vi "MOKO Graph.vi"() -> ()   [LabVIEW 2018]
uses:
  Lib/STM/Graph/MOKO_Graph_main_STM.ctl
  Lib/STM/Graph/MOKO_Graph_main_ITEM.ctl
  Lib/STM/Grafic/MOKO_Grafic_ITEM.ctl
  Lib/STM/Grafic/MOKO_Grafic_STM.ctl
  Buttons/Clear Graph Button.ctl
  MOKOGraphClusterIn.ctl
panel:
  out "XY Graph":cluster{"X":dbl, "Y":dbl}[](graph)
  in  "Cluster in":T1
  out "Screenshot indicator":bool
  in  "Base64 String":string
  in  "Screenshot":bool
  in  "Clear Graph":T2
  out "MOKO_Graph":refnum<queue>
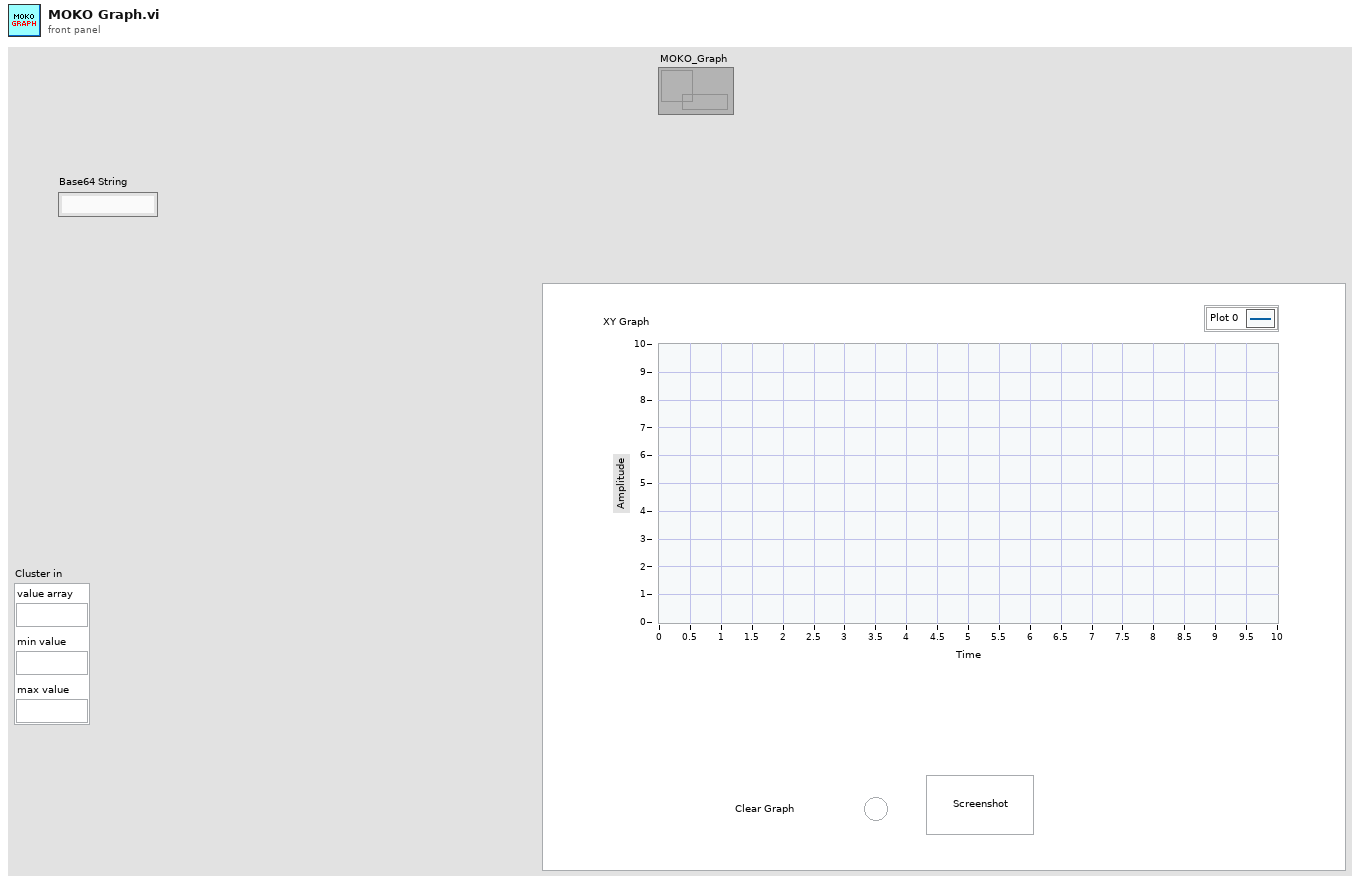
[diagram p1: front panel]
types:
  T1 = typedef "MOKOGraphClusterIn.ctl" = cluster{"value array":string, "min value":string, "max value":string}
  T2 = typedef "Clear Graph Button.ctl" = bool
  T3 = typedef "MOKO_Grafic_STM.ctl" = cluster{"main stm":T4, "data":string}
  T4 = typedef "MOKO_Grafic_ITEM.ctl" = enum16{"idle", "_____ LED STATE_____ ", "Write Graph", "Clear Graph", "Stop", "Screenshot"}
  T5 = typedef "MOKO_Graph_main_STM.ctl" = cluster{"main stm":T6, "data":string}
  T6 = typedef "MOKO_Graph_main_ITEM.ctl" = enum16{"idle", "Graph read", "Graph write"}
  T7 = typedef "imagedata.ctl" = cluster{"image type":i32, "image depth":i32, "image":u8[], "mask":u8[], "colors":u32[], "Rectangle":cluster{"left":i16, "top":i16, "right":i16, "bottom":i16}}
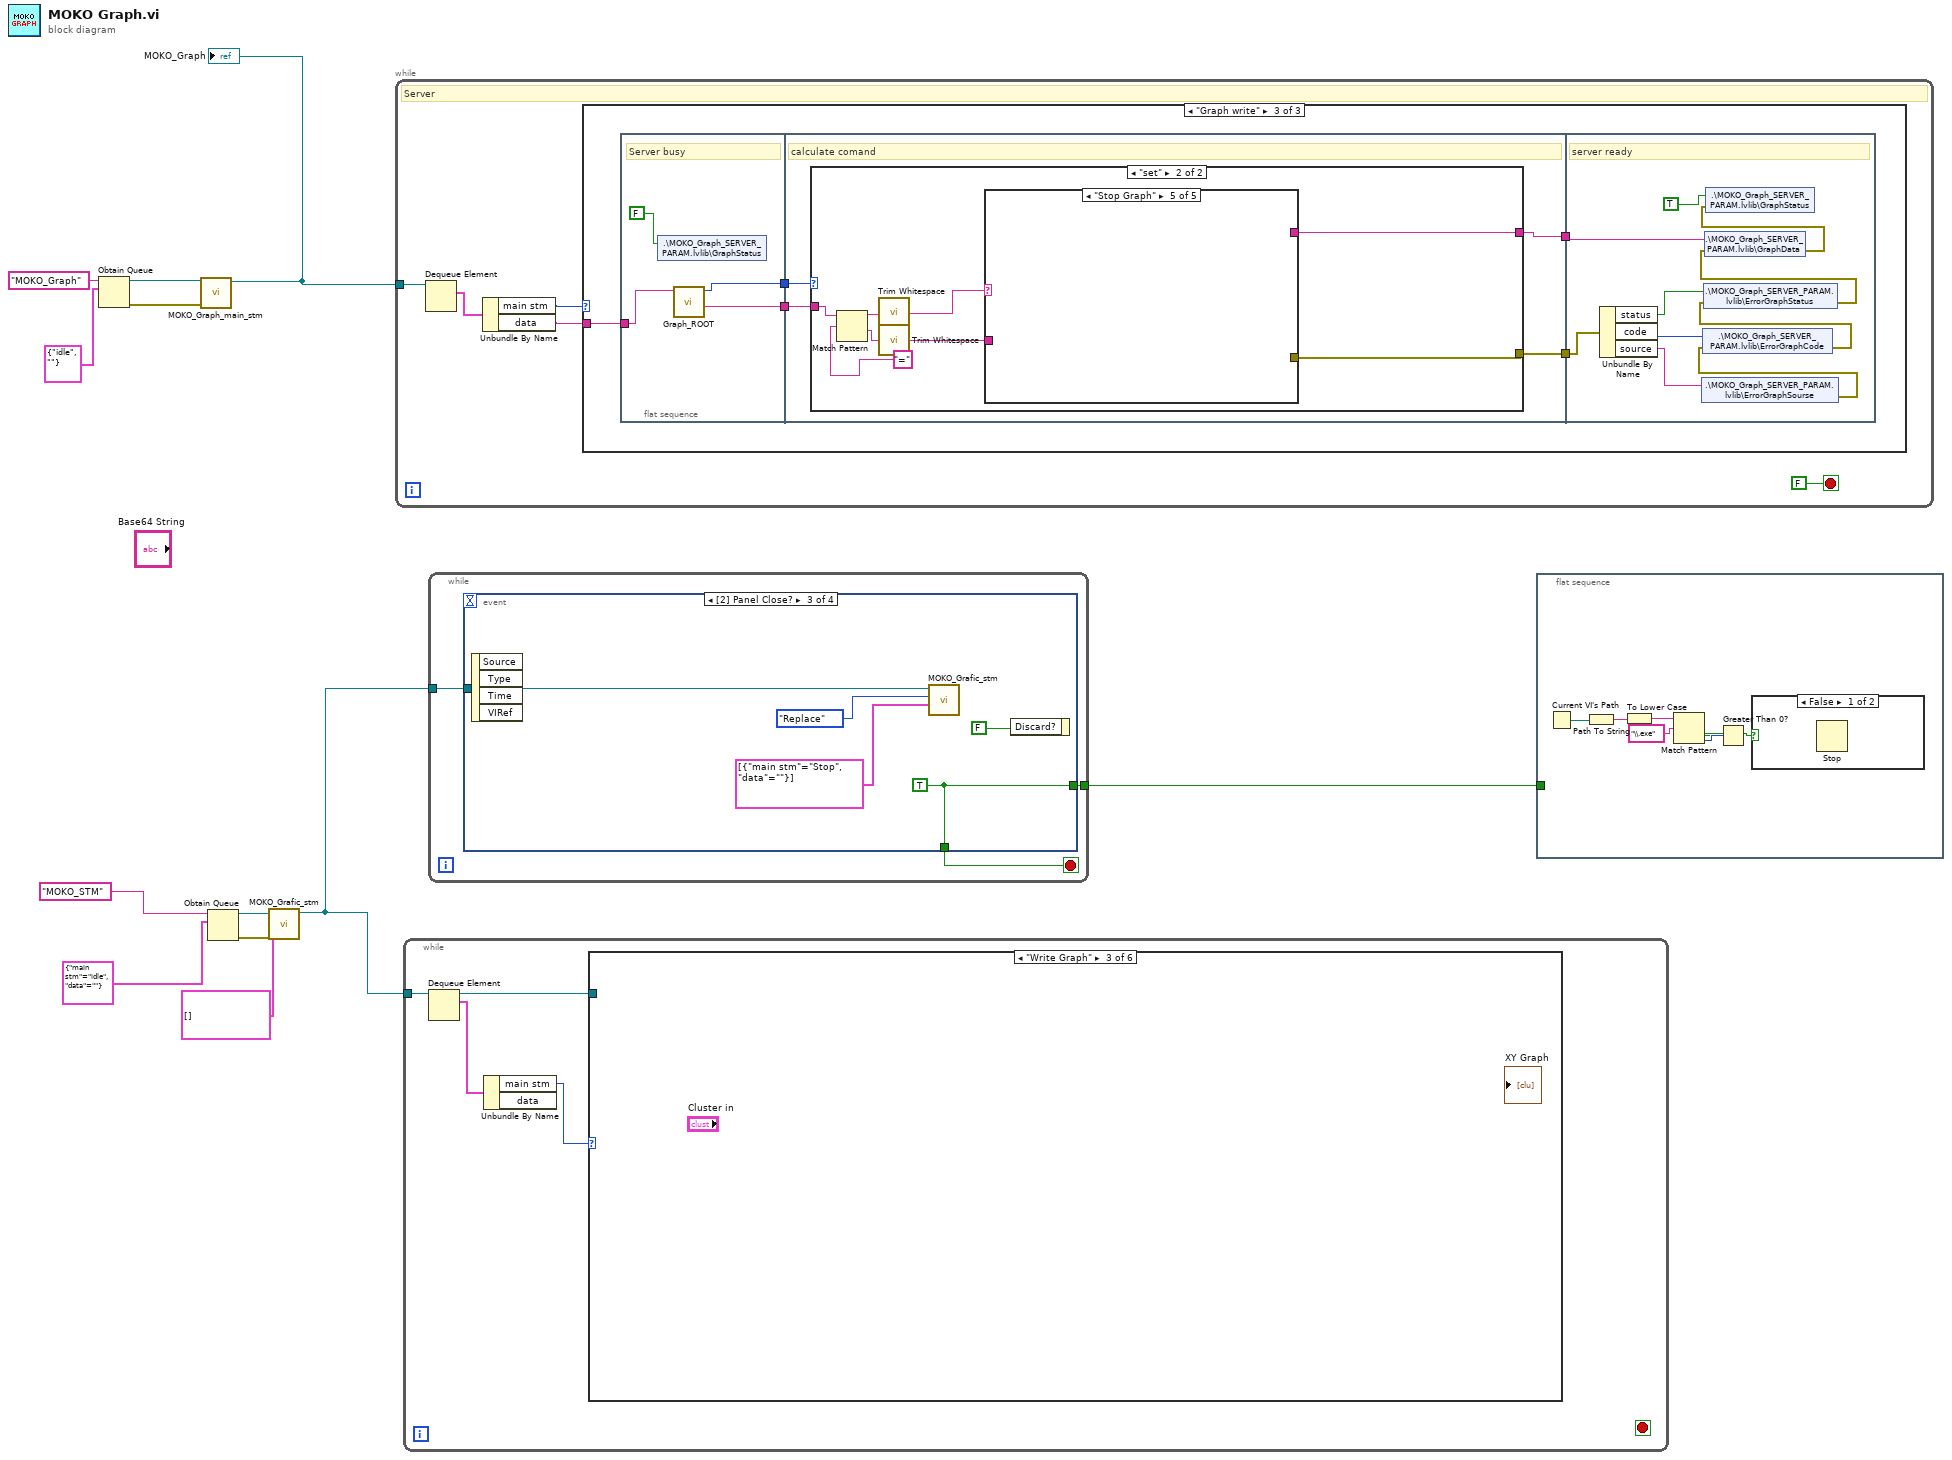
[diagram p0: block diagram]
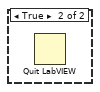
[diagram p2: hidden frame]
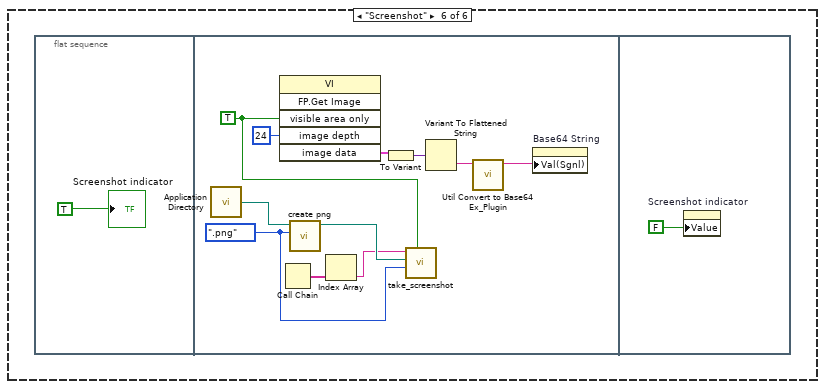
[diagram p7: hidden frame]
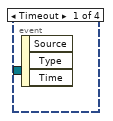
[diagram p8: hidden frame]
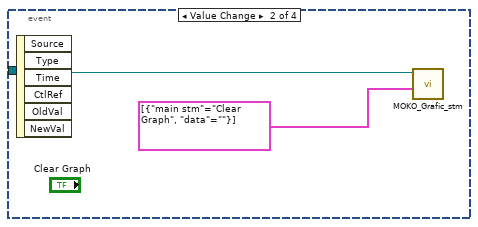
[diagram p9: hidden frame]
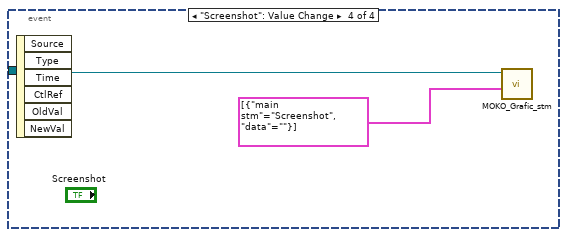
[diagram p10: hidden frame]
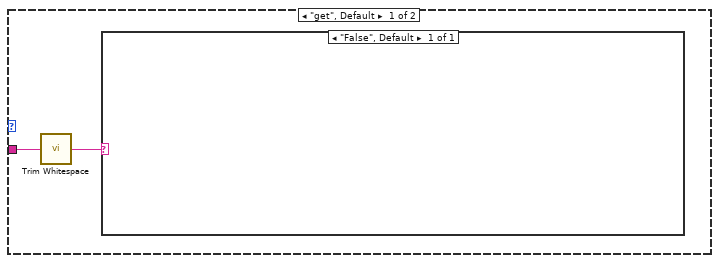
[diagram p13: hidden frame]
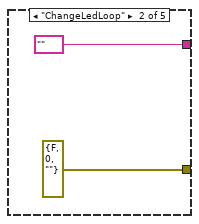
[diagram p15: hidden frame]
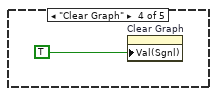
[diagram p17: hidden frame]
diagram:
  n1 = Obtain Queue(name (unnamed)="MOKO_Graph", element data type=T5 {"main stm"=enum."idle", "data"=""} ("MOKO_SE_STM")) -> (queue out=w10:refnum<queue>, error out=w9:errorcluster)  [unwired: 3 in, 1 out]
  n2 = call "MOKO_Graph_main_stm.vi"("error in"=w9, "queue in"=w10) -> ("queue out"=w8:refnum<queue>)  [unwired: 8 in, 1 out]
  "MOKO_Graph" <- w8
  n3 = Obtain Queue(name (unnamed)="MOKO_STM", element data type=T3 {"main stm"=enum."idle", "data"=""} ("MOKO_SE_STM")) -> (queue out=w6:refnum<queue>, error out=w5:errorcluster)  [unwired: 3 in, 1 out]
  n4 = call "MOKO_Grafic_stm.vi"("error in"=w5, "StateMachineSteps"=T3[] [], "queue in"=w6) -> ("queue out"=w4:refnum<queue>)  [unwired: 7 in, 1 out]
  n5 = while {
    tunnel: w8 -> [w16]
    stop <- FALSE stop-if-true
    # "Server"
    n6 = Dequeue Element(queue=w16) -> (element=w17:T5)  [unwired: 2 in, 3 out]
    n7 = Unbundle By Name(w17) -> ("main stm"=w15:T6, "data"=w14:string)
    n8 = case shown="\"Graph write\"" w15 {
      tunnel: w14 -> [_ _ w20]
      frame "idle", Default {
      }
      frame "Graph read" {
      }
      frame "Graph write" {
        n9 = flat-sequence {
          tunnel: w20 -> [w25]
          tunnel: [w24] -> w19
          tunnel: [w23] -> w18
          tunnel: [w27] -> w22
          tunnel: [w30] -> w21
          tunnel: w19 -> [w29]
          tunnel: w18 -> [w28]
          tunnel: w22 -> [w48]
          tunnel: w21 -> [w47]
          frame #0 {
            # "Server busy"
            n10 = shared-variable ".\\MOKO_Graph_SERVER_PARAM.lvlib\\GraphStatus"(FALSE) -> ()  [unwired: 1 in, 1 out]
            n11 = call "Graph_ROOT.vi"("data"=w25) -> ("command"=w23:string, "Mode out"=w24:enum16{"get", "set", "close", "Init", "Check"})  [unwired: 7 in, 2 out]
          }
          frame #1 {
            # "calculate comand"
            n12 = case shown="\"set\"" w29 {
              tunnel: [_ w40] -> w30
              tunnel: w28 -> [w32 w38]
              tunnel: [_ w33] -> w27
              frame "get", Default {
                n13 = call <vilib>:"Trim Whitespace.vi"("string"=w32) -> ("trimmed string"=w31:string)  [unwired: 1 in]
                n14 = case shown="\"False\", Default" w31 {
                  frame "False", Default {
                  }
                }
              }
              frame "set" {
                n15 = Match Pattern(string=w38, regular expression="=") -> (before substring=w36:string, after substring=w39:string)  [unwired: 1 in, 2 out]
                n16 = call <vilib>:"Trim Whitespace.vi"("string"=w36) -> ("trimmed string"=w35:string)  [unwired: 1 in]
                n17 = call <vilib>:"Trim Whitespace.vi"("string"=w39) -> ("trimmed string"=w34:string)  [unwired: 1 in]
                n18 = case shown="\"Stop Graph\"" w35 {
                  tunnel: [_ errorcluster {"status"=FALSE, "code"=0, "source"=""} ("error out") _ _ _] -> w40
                  tunnel: w34 -> [_ _ _ _ _]
                  tunnel: [_ "" _ _ _] -> w33
                  frame "False", Default {
                  }
                  frame "ChangeLedLoop" {
                  }
                  frame "Start Graph" {
                  }
                  frame "Clear Graph" {
                    n19 = property on="Clear Graph" class="Bool (strict)"("Val(Sgnl)"=TRUE) -> ()  [unwired: 2 in, 2 out]
                  }
                  frame "Stop Graph" {
                  }
                }
              }
            }
          }
          frame #2 {
            # "server ready"
            n20 = Unbundle By Name(w47) -> ("status"=w46:bool, "code"=w45:i32, "source"=w44:string)
            n21 = shared-variable ".\\MOKO_Graph_SERVER_PARAM.lvlib\\ErrorGraphSourse"(w44) -> (error out=w50:errorcluster)  [unwired: 1 in]
            n22 = shared-variable ".\\MOKO_Graph_SERVER_PARAM.lvlib\\ErrorGraphCode"(w45, error in=w50) -> (error out=w51:errorcluster)
            n23 = shared-variable ".\\MOKO_Graph_SERVER_PARAM.lvlib\\ErrorGraphStatus"(w46, error in=w51) -> (error out=w52:errorcluster)
            n24 = shared-variable ".\\MOKO_Graph_SERVER_PARAM.lvlib\\GraphData"(w48, error in=w52) -> (error out=w53:errorcluster)
            n25 = shared-variable ".\\MOKO_Graph_SERVER_PARAM.lvlib\\GraphStatus"(TRUE, error in=w53) -> ()  [unwired: 1 out]
          }
        }
      }
    }
  }
  n26 = while {
    tunnel: w4 -> [w57]
    stop <- _ stop-if-true
    n27 = Dequeue Element(queue=w57) -> (queue out=w55:refnum<queue>, element=w56:T3)  [unwired: 2 in, 2 out]
    n28 = Unbundle By Name(w56) -> ("main stm"=w54:T4)  [unwired: 1 out]
    n29 = case shown="\"Write Graph\"" w54 {
      tunnel: w55 -> [_ _ _ _ _ _]
      frame "idle", Default {
      }
      frame "_____ LED STATE_____ " {
      }
      frame "Write Graph" {
      }
      frame "Clear Graph" {
      }
      frame "Stop" {
      }
      frame "Screenshot" {
        n30 = flat-sequence {
          frame #0 {
            "Screenshot indicator" <- TRUE
          }
          frame #1 {
            w63 = TRUE ("Visible Area Only")
            w67 = enum32{".png", ".jpg", ".bmp"}.".png" ("IMG_FORMAT")
            n31 = call <vilib>:"Application Directory.vi"() -> ("Application Directory"=w69:path)
            n32 = invoke class="VI" method="FP.Get Image"("visible area only"=w63, "image depth"=24 ("Image Depth")) -> ("image data"=w61:T7)  [unwired: 4 in, 5 out]
            n33 = Call Chain() -> (call chain=w66:string[])
            n34 = call "create png.vi"("IMG_FORMAT"=w67, "base path"=w69) -> ("path"=w68:path)  [unwired: 8 in, 1 out]
            n35 = Index Array(array=w66) -> (element=w65:string)  [unwired: 1 in]
            n36 = To Variant(anything=w61) -> (Variant=w62:variant)
            n37 = call "take_screenshot.vi"("Visible area only? (f)"=w63, "IMG_FORMAT"=w67, "Image path"=w68, "vi path"=w65) -> ()  [unwired: 3 in, 2 out]
            n38 = Variant To Flattened String(Variant=w62) -> (data string=w60:string)  [unwired: 1 out]
            n39 = call "Util Convert to Base64 Ex_Plugin.vi"("String"=w60) -> ("Base64 String"=w59:string)  [unwired: 10 in]
            n40 = property on="Base64 String" class="Str"("Val(Sgnl)"=w59) -> ()  [unwired: 2 in, 2 out]
          }
          frame #2 {
            n41 = property on="Screenshot indicator" class="Bool (strict)"("Value"=FALSE) -> ()  [unwired: 2 in, 2 out]
          }
        }
      }
    }
  }
  n42 = while {
    tunnel: w4 -> [w73]
    tunnel: [w71] -> w2
    stop <- w72 stop-if-true
    n43 = event shown="[2] Panel Close?" {
      selector: _ -> [_ _ _ _]
      dyn-events: _ -> [_ _ _ _]
      timeout: _ -> [_ _ _ _]
      tunnel: w73 -> [_ w74 w80 w81]
      tunnel: [_ _ w76 _] -> w72
      tunnel: [_ _ w76 _] -> w71
      event Timeout {
        n44 = event-data() -> ()  [unwired: 1 in, 3 out]
      }
      event Value Change {
        n45 = event-data() -> ()  [unwired: 1 in, 6 out]
        n46 = call "MOKO_Grafic_stm.vi"("StateMachineSteps"=T3[] [{"main stm"=enum."Clear Graph", "data"=""}], "queue in"=w74) -> ()  [unwired: 8 in, 2 out]
      }
      event Panel Close? {
        w76 = TRUE
        n47 = event-data() -> ()  [unwired: 1 in, 4 out]
        n48 = call "MOKO_Grafic_stm.vi"("StateMachineSteps"=T3[] [{"main stm"=enum."Stop", "data"=""}], "FNs"=enum16{"Back", "Front", "Replace"}."Replace", "queue in"=w80) -> ()  [unwired: 7 in, 2 out]
        n49 = event-data("Discard?"=FALSE) -> ()  [unwired: 1 in, 1 out]
      }
      event "Screenshot": Value Change {
        n50 = event-data() -> ()  [unwired: 1 in, 6 out]
        n51 = call "MOKO_Grafic_stm.vi"("StateMachineSteps"=T3[] [{"main stm"=enum."Screenshot", "data"=""}], "queue in"=w81) -> ()  [unwired: 8 in, 2 out]
      }
    }
  }
  n52 = flat-sequence {
    tunnel: w2 -> [_]
    frame #0 {
      n53 = Current VI's Path() -> (path=w85:path)
      n54 = Path To String(path=w85) -> (string=w86:string)
      n55 = To Lower Case(string=w86) -> (all lower case string=w87:string)
      n56 = Match Pattern(string=w87, regular expression="\\.exe") -> (offset past match=w88:i32)  [unwired: 1 in, 3 out]
      n57 = Greater Than 0?(x=w88) -> (x > 0?=w84:bool)
      n58 = case shown="False" w84 {
        frame False {
          n59 = Stop() -> ()  [unwired: 1 in]
        }
        frame True {
          n60 = Quit LabVIEW() -> ()  [unwired: 1 in]
        }
      }
    }
  }
